vi "Pre Launch Init.vi"(11 "Measure Object in":refnum<class "Application Controller.lvclass">) -> (0 "error out":errorcluster, 3 "Measure Object out":refnum<class "Application Controller.lvclass">)   [LabVIEW 2018, in "Application Controller.lvclass"]
doc: "(<B>Filename</B>: Actor Framework.lvlib:Actor.lvclass:Pre Launch Init.vi)\n\nDefines behavior that occurs after the Launch Nested Actor method is invoked but before the actor's Actor Core method begins running.\n\nBy default, this method does nothing. A descendant class may override it to define behavior."
uses:
  Application Controller.lvclass
  Application Controller.lvclass/Application Controller.ctl
  Process Controller/Process Controller.lvclass
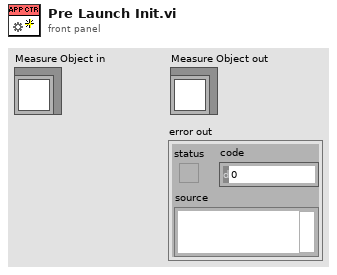
[diagram p1: front panel]
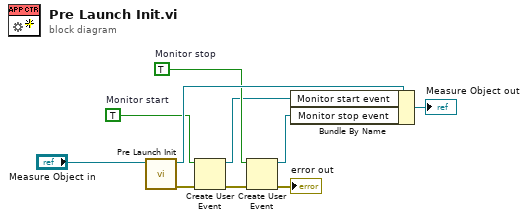
[diagram p0: block diagram]
diagram:
  w6 = TRUE  # Monitor stop
  w7 = TRUE  # Monitor start
  n1 = call-parent "Pre Launch Init.vi"("Measure Object in"="Measure Object in") -> ("error out"=w5:errorcluster, "Measure Object out"=w9:refnum<class "Application Controller.lvclass">)  [unwired: 9 in]
  n2 = Create User Event(user event datatype=w7, error in=w5) -> (user event=w1:refnum<user-event>, error out=w4:errorcluster)
  n3 = Create User Event(user event datatype=w6, error in=w4) -> (user event=w2:refnum<user-event>, error out=→"error out":errorcluster)
  n4 = Bundle By Name(cluster=w9, "Monitor start event"=w1, "Monitor stop event"=w2) -> (→"Measure Object out":refnum<class "Application Controller.lvclass">)
